vi "MSEncoder Case-23-LinearAmpScan.vi"(8 "error in (no error)":errorcluster, 9 "ParamValIn":variant, 11 "MSEncoder in":refnum<class "MSEncoder.lvclass">) -> (0 "error out":errorcluster, 3 "MSEncoder out":refnum<class "MSEncoder.lvclass">)   [LabVIEW 2018, in "MSEncoder.lvclass"]
uses:
  MSEncoder.lvclass
  Ctl/MSEditorParam linearAmpScan.ctl
  PublicSubVI/Ctl/MathieuEqParam.ctl
  MSEncoder.lvclass/MSEncoder.ctl
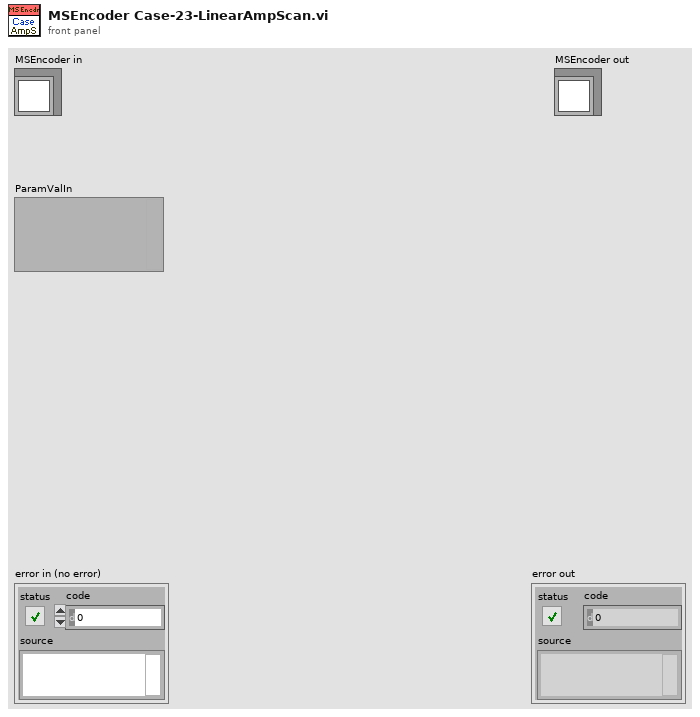
[diagram p1: front panel]
types:
  T1 = typedef "MSEditorParam linearAmpScan.ctl" = cluster{"auxWfmType":u8, "iauxCyc":dbl, "beta":dbl, "betaScale":dbl, "auxAmp":ext[], "auxPulse1":dbl[], "auxPulse2":dbl[], "auxPulseAmp":ext[], "time":ext, "amp":ext[], "continuous":bool}
  T2 = typedef "MathieuEqParam.ctl" = cluster{"mz(Th)":ext, "Amp(V)":ext, "Freq(Hz)":ext, "Beta":ext, "r_0 (mm)":ext, "z_0 (mm)":ext}
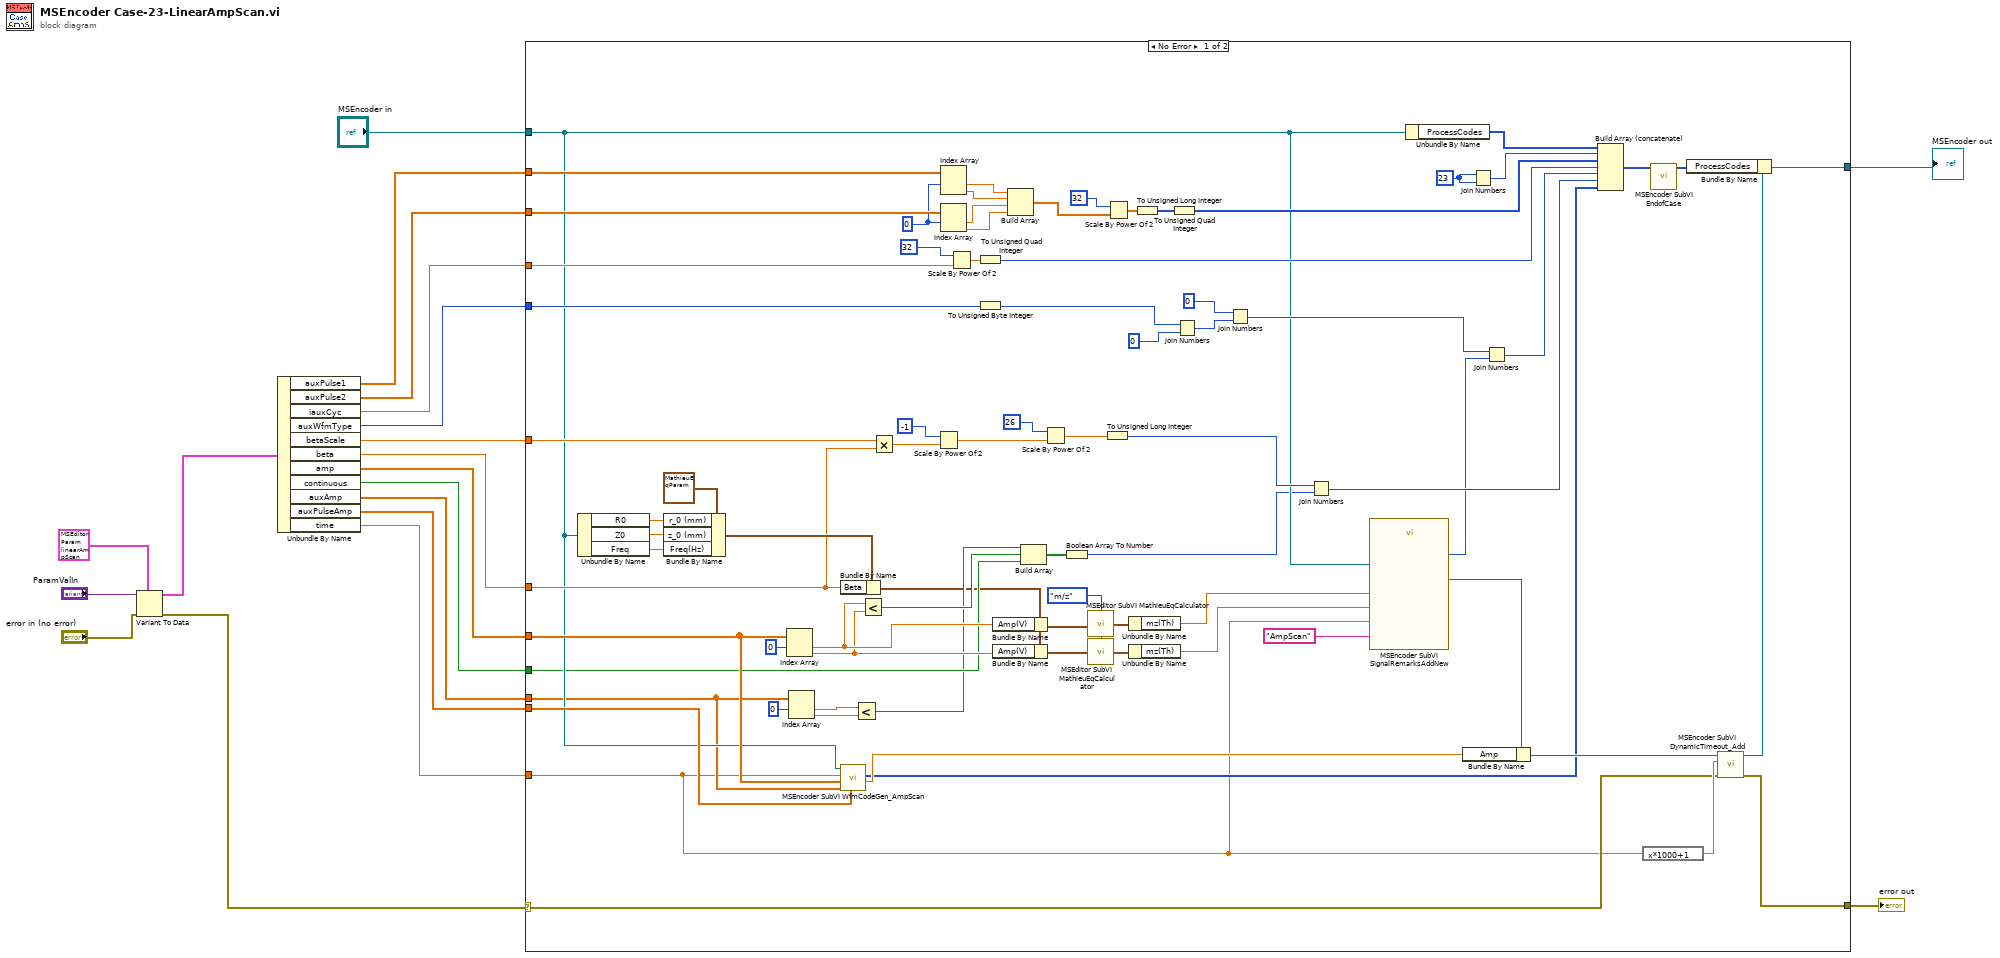
[diagram p0: block diagram]
diagram:
  n1 = Variant To Data(error in="error in (no error)", type=T1 {"auxWfmType"=0, "iauxCyc"=0.0, "beta"=0.0, "betaScale"=0.0, "auxAmp"=[], "auxPulse1"=[], "auxPulse2"=[], "auxPulseAmp"=[], "time"=0.0, "amp"=[], "continuous"=FALSE} ("linearAmpScan"), Variant="ParamValIn") -> (data=w5:T1, error out=w4:errorcluster)
  n2 = Unbundle By Name(w5) -> ("auxPulse1"=w1:dbl[], "auxPulse2"=w18:dbl[], "iauxCyc"=w17:dbl, "auxWfmType"=w16:u8, "betaScale"=w15:dbl, "beta"=w14:dbl, "amp"=w13:ext[], "continuous"=w3:bool, "auxAmp"=w12:ext[], "auxPulseAmp"=w11:ext[], "time"=w10:ext)
  n3 = case shown="No Error" w4 {
    selector: w4 -> [w44 w98]
    tunnel: "MSEncoder in" -> [w37 w97]
    tunnel: [w46 w98] -> w19
    tunnel: [w96 w97] -> w8
    tunnel: w1 -> [w90 _]
    tunnel: w18 -> [w89 _]
    tunnel: w17 -> [w88 _]
    tunnel: w16 -> [w87 _]
    tunnel: w15 -> [w86 _]
    tunnel: w14 -> [w85 _]
    tunnel: w13 -> [w39 _]
    tunnel: w12 -> [w29 _]
    tunnel: w11 -> [w38 _]
    tunnel: w10 -> [w22 _]
    tunnel: w3 -> [w32 _]
    frame No Error {
      w77 = u32 23
      w73 = 0 ("index")
      w80 = enum16{"m/z", "Volt", "Freq", "Beta"}."m/z" ("Target (Freq)")
      n4 = Unbundle By Name(w37) -> ("R0"=w95:ext, "Z0"=w94:ext, "Freq"=w93:ext)
      n5 = Bundle By Name(cluster=T2 {"mz(Th)"=0.0, "Amp(V)"=330.0, "Freq(Hz)"=0.0, "Beta"=1.0, "r_0 (mm)"=10.0, "z_0 (mm)"=7.0710678118654755} ("Parametres in"), "r_0 (mm)"=w95, "z_0 (mm)"=w94, "Freq(Hz)"=w93) -> (w91:T2)
      n6 = Index Array(array=w39, index #1=0 ("index")) -> (element #1=w41:ext, element #2=w40:ext)  [unwired: 1 in]
      n7 = Index Array(array=w29, index #1=0 ("index")) -> (element #1=w28:ext, element #2=w27:ext)  [unwired: 1 in]
      n8 = Bundle By Name(cluster=w91, "Beta"=w85) -> (w23:T2)
      n9 = call "MSEncoder SubVI WfmCodeGen_AmpScan.vi"("AuxPulses"=w38, "AuxAmp"=w29, "Amp"=w39, "Scan time"=w22, "MSEncoder in"=w37) -> ("Amp2"=w35:ext, "WfmCode"=w31:u64[])  [unwired: 5 in]
      n10 = Less?(x=w28, y=w27) -> (x < y?=w26:bool)
      n11 = Less?(x=w41, y=w40) -> (x < y?=w42:bool)
      n12 = Multiply(x=w86, y=w85) -> (x*y=w50:dbl)
      n13 = Scale By Power Of 2(n=i16 -1, x=w50) -> (x*2^n=w54:dbl)
      n14 = Index Array(array=w90, index #1=w73) -> (element #1=w70:dbl, element #2=w69:dbl)  [unwired: 1 in]
      n15 = Index Array(array=w89, index #1=w73) -> (element #1=w68:dbl, element #2=w67:dbl)  [unwired: 1 in]
      n16 = Scale By Power Of 2(n=i16 32, x=w88) -> (x*2^n=w75:dbl)
      n17 = To Unsigned Quad Integer(1:w75) -> (0:w61:u64)
      n18 = To Unsigned Byte Integer(number=w87) -> (unsigned 8bit integer=w49:u8)
      n19 = Bundle By Name(cluster=w23, "Amp(V)"=w41) -> (w71:T2)
      n20 = Bundle By Name(cluster=w23, "Amp(V)"=w40) -> (w84:T2)
      n21 = Build Array(w70, w69, w68, w67) -> (w65:dbl[])
      n22 = Build Array(w26, w42, w32) -> (w34:bool[])
      n23 = Scale By Power Of 2(n=i16 26, x=w54) -> (x*2^n=w53:dbl)
      n24 = Boolean Array To Number(Boolean array=w34) -> (number=w33:u32)
      n25 = call "MSEditor SubVI MathieuEqCalculator.vi"("Target (Freq)"=w80, "Parametres in"=w71) -> ("Parametres out"=w79:T2)  [unwired: 2 in]
      n26 = call "MSEditor SubVI MathieuEqCalculator.vi"("Target (Freq)"=w80, "Parametres in"=w84) -> ("Parametres out"=w72:T2)  [unwired: 2 in]
      n27 = To Unsigned Long Integer(number=w53) -> (unsigned 32bit integer=w52:u32)
      n28 = Scale By Power Of 2(n=i16 32, x=w65) -> (x*2^n=w64:dbl[])
      n29 = Unbundle By Name(w79) -> ("mz(Th)"=w21:ext)
      n30 = Unbundle By Name(w72) -> ("mz(Th)"=w20:ext)
      n31 = To Unsigned Long Integer(number=w64) -> (unsigned 32bit integer=w63:u32[])
      n32 = To Unsigned Quad Integer(1:w63) -> (0:w62:u64[])
      n33 = Join Numbers(hi=w49, lo=u8 0) -> ((hi.lo)=w60:u16)
      n34 = Join Numbers(hi=u16 0, lo=w60) -> ((hi.lo)=w58:u32)
      n35 = Join Numbers(hi=w52, lo=w33) -> ((hi.lo)=w51:u64)
      n36 = call "MSEncoder SubVI SignalRemarksAddNew.vi"("Label"="AmpScan", "Scan time"=w22, "mz 1"=w20, "mz 0"=w21, "MSEncoder in"=w37) -> ("Len"=w25:u32, "MSEncoder out"=w43:refnum<class "MSEncoder.lvclass">)  [unwired: 5 in]
      n37 = Unbundle By Name(w37) -> ("ProcessCodes"=w74:u64[])
      n38 = Bundle By Name(cluster=w43, "Amp"=w35) -> (w36:refnum<class "MSEncoder.lvclass">)
      n39 = Join Numbers(hi=w77, lo=w77) -> ((hi.lo)=w83:u64)
      n40 = Join Numbers(hi=w58, lo=w25) -> ((hi.lo)=w57:u64)
      n41 = Build Array (concatenate)(w74, w83, w62, w61, w57, w51, w31) -> (w82:u64[])
      n42 = expression code="x*1000+1"(w22) -> (w48:ext)
      n43 = call "MSEncoder SubVI EndofCase.vi"("Case codes"=w82) -> ("Case codes with end"=w81:u64[])  [unwired: 9 in, 1 out]
      n44 = call "MSEncoder SubVI DynamicTimeout_Add.vi"("error in (no error)"=w44, "Timeout_ms"=w48, "MSEncoder"=w36) -> ("error out"=w46:errorcluster, "MSEncoder"=w47:refnum<class "MSEncoder.lvclass">)  [unwired: 7 in]
      n45 = Bundle By Name(cluster=w47, "ProcessCodes"=w81) -> (w96:refnum<class "MSEncoder.lvclass">)
    }
    frame Error {
    }
  }
  "error out" <- w19
  "MSEncoder out" <- w8
